vi "Periodic Tasks.vi"() -> ()   [LabVIEW 2012]
doc: "This VI runs in parallel to other tasks. It can contain as many user-defined periodic loops as you need. These can carry out PID or other sorts of timed response."
uses:
  <vilib>/Rock Robotics/SystemInterfaces/Utilities/FPGA_UtilitiesLED Source.ctl
  <vilib>/Rock Robotics/SystemInterfaces/Utilities/FPGA_UtilitiesLED State.ctl
  Robot Global Data.vi
panel:
  in  "FlipUp":bool
  in  "Use DS Data":bool
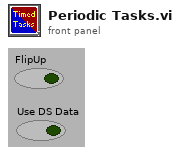
[diagram p1: front panel]
types:
  T1 = typedef "FPGA_UtilitiesLED State.ctl" = enum16{"Off", "On", "Toggle"}
  T2 = typedef "FPGA_UtilitiesLED Source.ctl" = enum16{"User LED", "FPGA LED"}
  T3 = cluster{"Case":dbl, "VisionTrack":bool, "ShootEnableWheels":bool, "Shoot":bool, "ManualExtend":dbl, "ManualRotate":dbl, "YCoord":dbl, "FlipUp":bool, "RotDeadband":dbl, "ExtDeadband":dbl, "ExtPOT":dbl, "RotPOT":dbl, "WheelFSpd":dbl, "WheelBSpd":dbl, "ServoPositions":cluster{"FlipperLeftUp":dbl, "FlipperLeftDown":dbl, "FlipperRightUp":dbl, "FlipperRightDown":dbl, "KickerLeftBack":dbl, "KickerLeftForward":dbl, "KickerRightBack":dbl, "KickerRightForward":dbl}, "POTPositions":cluster{"Setpoint 1":dbl, "Setpoint 2":dbl, "Setpoint 3":dbl, "Setpoint 4":dbl, "RotLow":dbl, "RotHigh":dbl, "ExtLow":dbl, "ExtHigh":dbl}, "ClimberHooked":bool}
  T4 = cluster{"FlipperLeftUp":dbl, "FlipperLeftDown":dbl, "FlipperRightUp":dbl, "FlipperRightDown":dbl, "KickerLeftBack":dbl, "KickerLeftForward":dbl, "KickerRightBack":dbl, "KickerRightForward":dbl}
  T5 = cluster{"Setpoint 1":dbl, "Setpoint 2":dbl, "Setpoint 3":dbl, "Setpoint 4":dbl, "RotLow":dbl, "RotHigh":dbl, "ExtLow":dbl, "ExtHigh":dbl}
  T6 = typedef "WPI_AnalogChannelDevRef.ctl" = cluster{"DevStatus":errorcluster, "Analog Module":T7, "Analog Channel":T8}
  T7 = typedef "FPGA_TypedefAnalogModule.ctl" = enum16{"Analog Module 1", "Analog Module 2"}
  T8 = typedef "FPGA_AIChannel.ctl" = enum8{"AI 1", "AI 2", "AI 3", "AI 4", "AI 5", "AI 6", "AI 7", "AI 8", "Invalid"}
  T9 = typedef "WPI_RelayValue.ctl" = enum16{"Off", "On", "Forward", "Reverse"}
  T10 = cluster{"Case":dbl, "Extension":dbl, "Rotation":dbl, "WheelF":dbl, "WheelB":dbl, "Left Kicker":dbl, "Right Kicker":dbl, "Left Flipper":dbl, "Right Flipper":dbl, "Lights":T9}
  T11 = typedef "WPI_GyroDevRef.ctl" = cluster{"DevStatus":errorcluster, "Analog Module":T7, "Analog Channel":T8, "Offset":dbl, "Gain (VoltsPerDegree/Second)":dbl}
  T12 = typedef "WPI_EncoderDevRef.ctl" = cluster{"DevStatus":errorcluster, "EncoderIndex":T13, "CounterIndex":T14, "DistancePerCount":dbl, "Decoding Type":T15}
  T13 = typedef "FPGA_EncoderIdx.ctl" = enum8{"Enc 0", "Enc 1", "Enc 2", "Enc 3", "Invalid"}
  T14 = typedef "FPGA_CounterCtrSystemIndex.ctl" = enum8{"Ctr 0", "Ctr 1", "Ctr 2", "Ctr 3", "Ctr 4", "Ctr 5", "Ctr 6", "Ctr 7", "Invalid"}
  T15 = typedef "WPI_EncoderType.ctl" = enum16{"1x", "2x", "4x"}
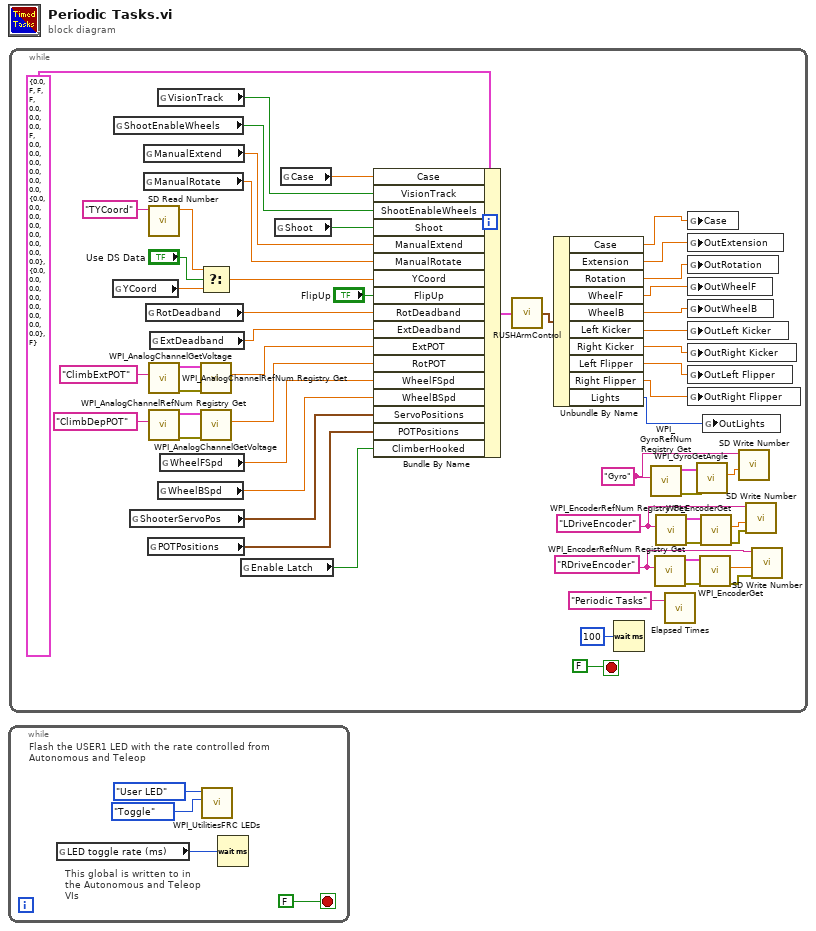
[diagram p0: block diagram]
diagram:
  n1 = while {
    stop <- FALSE stop-if-true
    # "This global is written to in the Autonomous and Teleop VIs"
    # "Flash the USER1 LED with the rate controlled from Autonomous and Teleop"
    n2 = global read "Robot Global Data.vi" "LED toggle rate (ms)"() -> (w1:u32)
    n3 = call <vilib>:"WPI_UtilitiesFRC LEDs.vi"("State"=FPGA_UtilitiesLED_State."Toggle", "LED Type"=FPGA_UtilitiesLED_Source."User LED") -> ()  [unwired: 1 in, 9 out]
    n4 = Wait (ms)(milliseconds to wait=w1) -> ()  [unwired: 1 out]
  }
  n5 = while {
    stop <- FALSE stop-if-true
    w13 = "RDriveEncoder" ("refnum name")
    w9 = "LDriveEncoder" ("refnum name")
    w7 = "Gyro" ("refnum name")
    n6 = global read "Robot Global Data.vi" "YCoord"() -> (w27:dbl)
    n7 = global read "Robot Global Data.vi" "ShootEnableWheels"() -> (w42:bool)
    n8 = global read "Robot Global Data.vi" "ShooterServoPos"() -> (w34:T4)
    n9 = global read "Robot Global Data.vi" "ManualExtend"() -> (w40:dbl)
    n10 = global read "Robot Global Data.vi" "ManualRotate"() -> (w39:dbl)
    n11 = global read "Robot Global Data.vi" "RotDeadband"() -> (w38:dbl)
    n12 = global read "Robot Global Data.vi" "POTPositions"() -> (w33:T5)
    n13 = call <vilib>:"SD Read Number.vi"("Name"="TYCoord") -> ("Numeric"=w28:dbl)  [unwired: 8 in, 2 out]
    n14 = call <vilib>:"WPI_AnalogChannelRefNum Registry Get.vi"("refnum name"="ClimbExtPOT") -> ("error out"=w56:errorcluster, "AIDeviceRef"=w55:T6)  [unwired: 9 in]
    n15 = call <vilib>:"WPI_AnalogChannelRefNum Registry Get.vi"("refnum name"="ClimbDepPOT") -> ("error out"=w50:errorcluster, "AIDeviceRef"=w49:T6)  [unwired: 9 in]
    n16 = global read "Robot Global Data.vi" "ExtDeadband"() -> (w37:dbl)
    n17 = global read "Robot Global Data.vi" "VisionTrack"() -> (w43:bool)
    n18 = global read "Robot Global Data.vi" "WheelBSpd"() -> (w35:dbl)
    n19 = global read "Robot Global Data.vi" "WheelFSpd"() -> (w36:dbl)
    n20 = Select(t=w28, s="Use DS Data", f=w27) -> (s? t:f=w25:dbl)
    n21 = call <vilib>:"WPI_AnalogChannelGetVoltage.vi"("error in (no error)"=w56, "AIDeviceRef"=w55) -> ("Voltage"=w30:dbl)  [unwired: 7 in, 2 out]
    n22 = call <vilib>:"WPI_AnalogChannelGetVoltage.vi"("error in (no error)"=w50, "AIDeviceRef"=w49) -> ("Voltage"=w29:dbl)  [unwired: 7 in, 2 out]
    n23 = global read "Robot Global Data.vi" "Enable Latch"() -> (w5:bool)
    n24 = global read "Robot Global Data.vi" "Shoot"() -> (w41:bool)
    n25 = global read "Robot Global Data.vi" "Case"() -> (w44:dbl)
    n26 = Bundle By Name(cluster=T3 {"Case"=0.0, "VisionTrack"=FALSE, "ShootEnableWheels"=FALSE, "Shoot"=FALSE, "ManualExtend"=0.0, "ManualRotate"=0.0, "YCoord"=0.0, "FlipUp"=FALSE, "RotDeadband"=0.0, "ExtDeadband"=0.0, "ExtPOT"=0.0, "RotPOT"=0.0, "WheelFSpd"=0.0, "WheelBSpd"=0.0, "ServoPositions"={"FlipperLeftUp"=0.0, "FlipperLeftDown"=0.0, "FlipperRightUp"=0.0, "FlipperRightDown"=0.0, "KickerLeftBack"=0.0, "KickerLeftForward"=0.0, "KickerRightBack"=0.0, "KickerRightForward"=0.0}, "POTPositions"={"Setpoint 1"=0.0, "Setpoint 2"=0.0, "Setpoint 3"=0.0, "Setpoint 4"=0.0, "RotLow"=0.0, "RotHigh"=0.0, "ExtLow"=0.0, "ExtHigh"=0.0}, "ClimberHooked"=FALSE} ("In Cluster"), "Case"=w44, "VisionTrack"=w43, "ShootEnableWheels"=w42, "Shoot"=w41, "ManualExtend"=w40, "ManualRotate"=w39, "YCoord"=w25, "FlipUp"="FlipUp", "RotDeadband"=w38, "ExtDeadband"=w37, "ExtPOT"=w30, "RotPOT"=w29, "WheelFSpd"=w36, "WheelBSpd"=w35, "ServoPositions"=w34, "POTPositions"=w33, "ClimberHooked"=w5) -> (w46:T3)
    n27 = call "RUSHArmControl.vi"("In Cluster"=w46) -> ("Out Cluster"=w45:T10)
    n28 = Unbundle By Name(w45) -> ("Case"=w24:dbl, "Extension"=w23:dbl, "Rotation"=w22:dbl, "WheelF"=w21:dbl, "WheelB"=w20:dbl, "Left Kicker"=w19:dbl, "Right Kicker"=w18:dbl, "Left Flipper"=w17:dbl, "Right Flipper"=w16:dbl, "Lights"=w6:T9)
    n29 = Wait (ms)(milliseconds to wait=u32 100) -> ()  [unwired: 1 out]
    n30 = call <vilib>:"WPI_GyroRefNum Registry Get.vi"("refnum name"=w7) -> ("error out"=w57:errorcluster, "GyroDevRef"=w58:T11)  [unwired: 9 in]
    n31 = call <vilib>:"WPI_EncoderRefNum Registry Get.vi"("refnum name"=w13) -> ("error out"=w52:errorcluster, "EncoderDevRef"=w51:T12)  [unwired: 9 in]
    n32 = call <vilib>:"WPI_EncoderRefNum Registry Get.vi"("refnum name"=w9) -> ("error out"=w53:errorcluster, "EncoderDevRef"=w54:T12)  [unwired: 9 in]
    n33 = call "Elapsed Times.vi"("Call Name"="Periodic Tasks") -> ()  [unwired: 2 in, 1 out]
    n34 = global write "Robot Global Data.vi" "Case"(w24) -> ()
    n35 = global write "Robot Global Data.vi" "OutExtension"(w23) -> ()
    n36 = global write "Robot Global Data.vi" "OutRotation"(w22) -> ()
    n37 = global write "Robot Global Data.vi" "OutWheelF"(w21) -> ()
    n38 = global write "Robot Global Data.vi" "OutWheelB"(w20) -> ()
    n39 = global write "Robot Global Data.vi" "OutLeft Kicker"(w19) -> ()
    n40 = global write "Robot Global Data.vi" "OutRight Kicker"(w18) -> ()
    n41 = global write "Robot Global Data.vi" "OutLeft Flipper"(w17) -> ()
    n42 = global write "Robot Global Data.vi" "OutRight Flipper"(w16) -> ()
    n43 = call <vilib>:"WPI_GyroGetAngle.vi"("error in (no error)"=w57, "GyroDevRef"=w58) -> ("Angle"=w8:dbl)  [unwired: 6 in, 3 out]
    n44 = call <vilib>:"WPI_EncoderGet.vi"("error in (no error)"=w52, "EncoderDevRef"=w51) -> ("error out"=w10:errorcluster, "Distance"=w14:dbl)  [unwired: 4 in, 4 out]
    n45 = call <vilib>:"WPI_EncoderGet.vi"("error in (no error)"=w53, "EncoderDevRef"=w54) -> ("error out"=w12:errorcluster, "Distance"=w11:dbl)  [unwired: 4 in, 4 out]
    n46 = global write "Robot Global Data.vi" "OutLights"(w6) -> ()
    n47 = call <vilib>:"SD Write Number.vi"("Numeric"=w8, "Name"=w7) -> ()  [unwired: 8 in, 2 out]
    n48 = call <vilib>:"SD Write Number.vi"("error in"=w12, "Numeric"=w11, "Name"=w9) -> ()  [unwired: 7 in, 2 out]
    n49 = call <vilib>:"SD Write Number.vi"("error in"=w10, "Numeric"=w14, "Name"=w13) -> ()  [unwired: 7 in, 2 out]
  }
